vi "2526 Initial Connect.vi"(8 "error in (no error)":errorcluster, 10 "JSONCluster":T1, 11 "IVI Refnum in":refnum<k15>) -> (0 "error out":errorcluster, 2 "Scan List Channels":string[](array[string]), 3 "IVI Refnum out":refnum<k15>)   [LabVIEW 2019, in "SupportVIs.lvlib"]
uses:
  SupportVIs.lvlib
  JSONCluster.ctl
  <instrlib>/niSwitch/niSwitch.llb/niSwitch Connect Channels (Single).vi
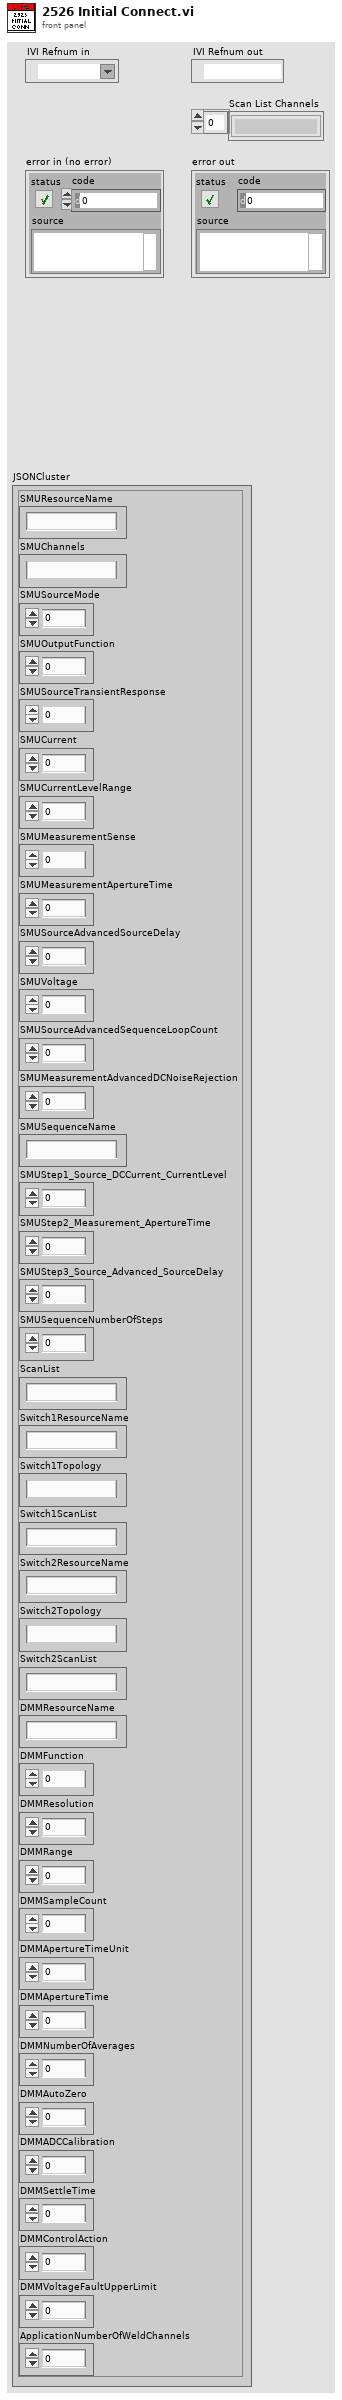
[diagram p1: front panel]
types:
  T1 = typedef "JSONCluster.ctl" = cluster{"SMUResourceName":string, "SMUChannels":string, "SMUSourceMode":i32, "SMUOutputFunction":i32, "SMUSourceTransientResponse":i32, "SMUCurrent":dbl, "SMUCurrentLevelRange":dbl, "SMUMeasurementSense":i32, "SMUMeasurementApertureTime":dbl, "SMUSourceAdvancedSourceDelay":dbl, "SMUVoltage":dbl, "SMUSourceAdvancedSequenceLoopCount":i32, "SMUMeasurementAdvancedDCNoiseRejection":i32, "SMUSequenceName":string, "SMUStep1_Source_DCCurrent_CurrentLevel":i32, "SMUStep2_Measurement_ApertureTime":i32, "SMUStep3_Source_Advanced_SourceDelay":i32, "SMUSequenceNumberOfSteps":i32, "ScanList":string, "Switch1ResourceName":string, "Switch1Topology":string, "Switch1ScanList":string, "Switch2ResourceName":string, "Switch2Topology":string, "Switch2ScanList":string, "DMMResourceName":string, "DMMFunction":i32, "DMMResolution":dbl, "DMMRange":dbl, "DMMSampleCount":i32, "DMMApertureTimeUnit":i32, "DMMApertureTime":dbl, "DMMNumberOfAverages":i32, "DMMAutoZero":i32, "DMMADCCalibration":i32, "DMMSettleTime":dbl, "DMMControlAction":i32, "DMMVoltageFaultUpperLimit":dbl, "ApplicationNumberOfWeldChannels":i32}
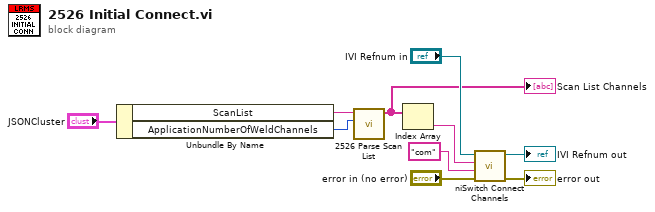
[diagram p0: block diagram]
diagram:
  n1 = Unbundle By Name("JSONCluster") -> ("ScanList"=w3:string, "ApplicationNumberOfWeldChannels"=w1:i32)
  n2 = call "2526 Parse Scan List.vi"("ApplicationNumberOfWeldChannels"=w1, "MUX Input String"=w3) -> ("Channel Array"=w2:string[])  [unwired: 9 in]
  "Scan List Channels" <- w2
  n3 = Index Array(array=w2) -> (element=w7:string)  [unwired: 1 in]
  n4 = call-poly <instrlib>:"niSwitch Connect Channels.vi"("error in (no error)"="error in (no error)", "channel 2"="com", "channel 1"=w7, "instrument handle"="IVI Refnum in") -> ("error out"=→"error out":errorcluster, "instrument handle out"=→"IVI Refnum out":refnum<k15>)  [unwired: 6 in]
